vi "_Register Group.vi"(6 "EventLogging":refnum<class "EventLoggingService.lvclass">, 8 "error in (no error)":errorcluster, 10 "Group":refnum<class "Group.lvclass">, 11 "Loop Data In":T1) -> (0 "error out":errorcluster, 3 "Loop Data":T1)   [LabVIEW 2020, in "Vecto.lvlib" / "RemoteDataService.lvclass"]
uses:
  RemoteDataService.lvclass
  Loop Data.ctl
  SequenceCountService/SequenceCountService.lvclass
  ChannelService/ChannelService.lvclass
  Published Group.ctl
  Packet.ctl
  lv-protoc/LV-Proto/Message/Message.lvclass
  Group Data Type.ctl
  Subscription.ctl
  Subscription Info.ctl
  SubscribedDataHandler/SubscribedDataHandler.lvclass
  VectoConfig/Telemetry Config.ctl
  VectoConfig/Telemetry Routing.ctl
  VectoConfig/Endpoint.ctl
  Group/Group.lvclass
  EventLoggingService/EventLoggingService.lvclass
  Event Level.ctl
  Group/Group.lvclass/Group.ctl
  Group Config/Group Config.lvclass/Group Config.ctl
  EventLoggingService/EventLoggingService.lvclass/EventLoggingService.ctl
  EventLogHandler/EventLogHandler.lvclass
  RemoteDataService.lvclass/RemoteDataService.ctl
  Group Config/Group Config.lvclass
  Vecto.lvlib
  VectoConfig/VectoConfig.lvlib
  IP Resolver/IP Resolver.lvclass
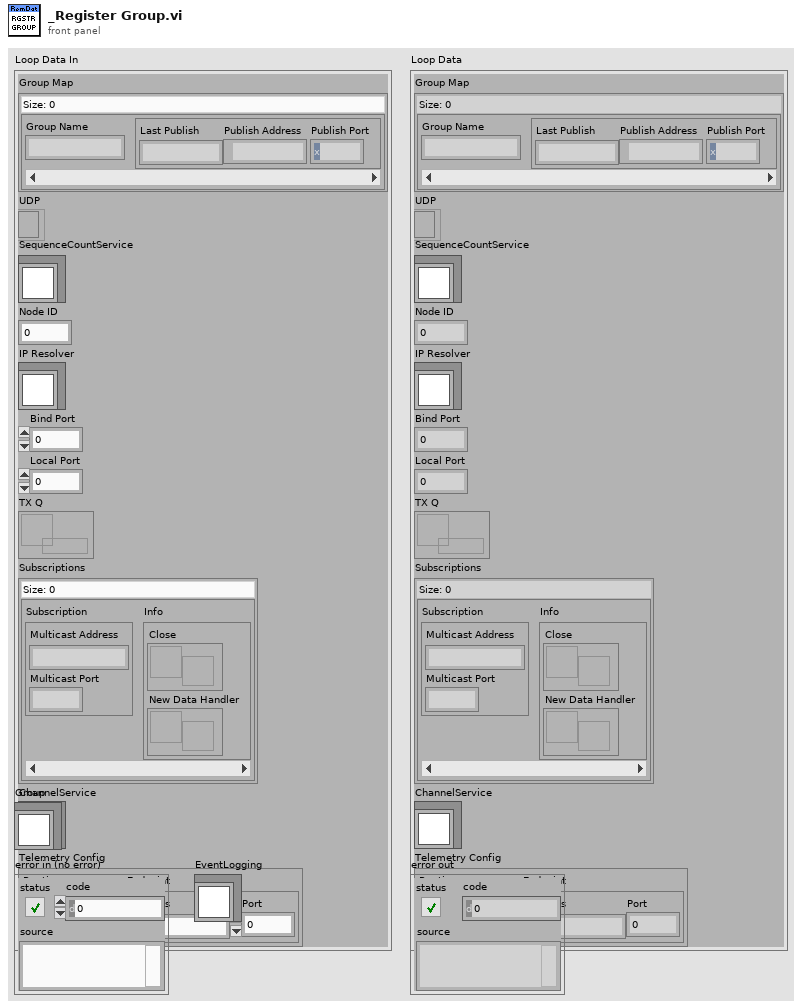
[diagram p1: front panel]
types:
  T1 = typedef "Vecto.lvlib/RemoteDataService.lvclass/Loop Data.ctl" = cluster{"Group Map":map{string, T2}, "UDP":refnum<k16>, "SequenceCountService":refnum<class "SequenceCountService.lvclass">, "Node ID":u32, "IP Resolver":refnum<class "IP Resolver.lvclass">, "Bind Port":u16, "Local Port":u16, "TX Q":refnum<queue>, "Subscriptions":map{T3, T4}, "ChannelService":refnum<class "ChannelService.lvclass">, "Telemetry Config":T5}
  T2 = typedef "Vecto.lvlib/RemoteDataService.lvclass/Published Group.ctl" = cluster{"Last Publish":dbl, "Publish Address":u32, "Publish Port":u16}
  T3 = typedef "Vecto.lvlib/RemoteDataService.lvclass/Subscription.ctl" = cluster{"Multicast Address":string, "Multicast Port":u16}
  T4 = typedef "Vecto.lvlib/RemoteDataService.lvclass/Subscription Info.ctl" = cluster{"Close":refnum<user-event>, "New Data Handler":refnum<user-event>}
  T5 = typedef "VectoConfig.lvlib/Telemetry Config.ctl" = cluster{"Routing":T6, "Endpoint":T7}
  T6 = typedef "VectoConfig.lvlib/Telemetry Routing.ctl" = enum16{"Multicast", "Unicast"}
  T7 = typedef "VectoConfig.lvlib/Endpoint.ctl" = cluster{"Address":string, "Port":u16}
  T8 = typedef "Vecto.lvlib/Event Level.ctl" = enum16{"Debug", "Info", "Warning", "Error"}
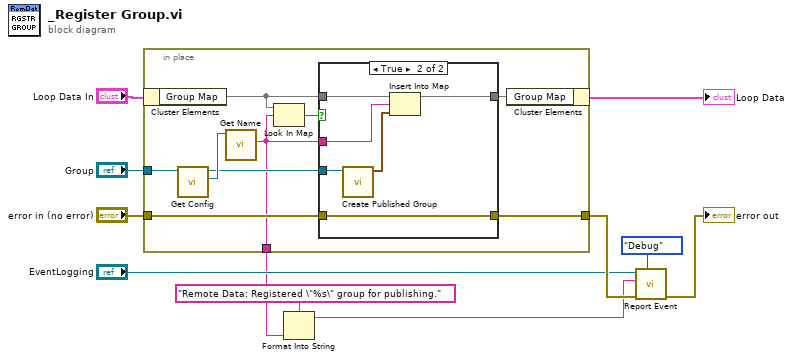
[diagram p0: block diagram]
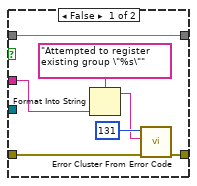
[diagram p2: hidden frame]
diagram:
  n1 = in-place {
    in-place-border: "Group" -> [w20]
    in-place-border: "error in (no error)" -> [w15]
    in-place-border: [w13] -> w11
    in-place-border: [w12] -> w3
    n2 = in-place-cluster #1("Loop Data In") -> ("Group Map"=w17:map{string, T2})
    n3 = call "Get Config.vi"("Group in"=w20) -> ("Config"=w19:refnum<class "Group Config.lvclass">, "Group out"=w16:refnum<class "Group.lvclass">)  [unwired: 8 in, 1 out]
    n4 = call "Get Name.vi"("Group Config in"=w19) -> ("Name"=w12:string)  [unwired: 8 in, 2 out]
    n5 = Look In Map(map=w17, key=w12) -> (key not found?=w18:bool)  [unwired: 1 in, 1 out]
    n6 = case shown="True" w18 {
      tunnel: w17 -> [w27 w31]
      tunnel: w16 -> [_ w29]
      tunnel: w12 -> [w24 w32]
      tunnel: w15 -> [w26 w33]
      tunnel: [w27 w30] -> w14
      tunnel: [w21 w33] -> w13
      frame False {
        n7 = Format Into String(format string="Attempted to register existing group \"%s\"", w24) -> (resulting string=w22:string)  [unwired: 2 in, 1 out]
        n8 = call <vilib>:"Error Cluster From Error Code.vi"("error in (no error)"=w26, "error message (\"\")"=w22, "error code (0)"=131) -> ("error out"=w21:errorcluster)  [unwired: 6 in]
      }
      frame True {
        n9 = call "Create Published Group.vi"("Group"=w29) -> ("Published Group"=w28:T2)  [unwired: 10 in]
        n10 = Insert Into Map(map in=w31, key=w32, value=w28) -> (map out=w30:map{string, T2})  [unwired: 2 out]
      }
    }
    n11 = in-place-cluster #1("Group Map"=w14) -> (→"Loop Data":T1)
  }
  n12 = Format Into String(format string="Remote Data: Registered \"%s\" group for publishing.", w3) -> (resulting string=w1:string)  [unwired: 2 in, 1 out]
  n13 = call "Report Event.vi"("Event Level (Info)"=Event_Level."Debug", "error in (no error)"=w11, "Message"=w1, "EventLoggingService in"="EventLogging") -> ("error out"=→"error out":errorcluster)  [unwired: 6 in, 1 out]
